vi "MySubsystem_Cals_Load.vi"(8 "error in":errorcluster, 11 "Subsystem":string="MySubsystem") -> ()   [LabVIEW 2020]
uses:
  MySubsystem_Global.vi
panel:
  out "Cals/MySubsystem/DblVariable1":dbl
  out "error out":errorcluster
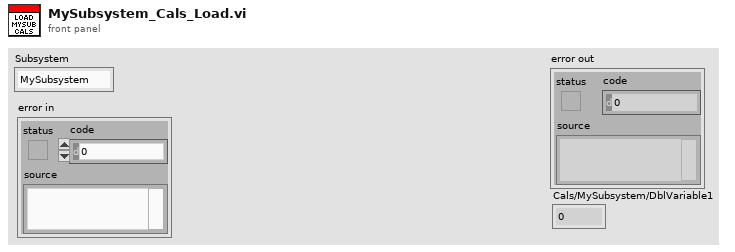
[diagram p1: front panel]
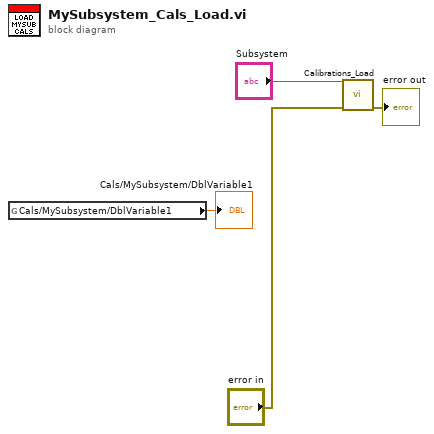
[diagram p0: block diagram]
diagram:
  n1 = global read "MySubsystem_Global.vi" "Cals/MySubsystem/DblVariable1"() -> (→"Cals/MySubsystem/DblVariable1":dbl)
  n2 = call "Calibrations_Load.vi"("error in"="error in", "Subsystem"="Subsystem") -> ("error out"=→"error out":errorcluster)  [unwired: 9 in]
